vi "generate limit circle.vi"(8 "Radius Limit (mm)":dbl, 9 "Location Description":string, 10 "NewVal":T2 {"List of locations"."Position"."Position Y" format="%#.3f"; "List of locations"."Position"."Position X" format="%#.3f"}, 11 "Device Description":string) -> (2 "Center location":T1 {"Position"."Position Y" format="%#.3f"; "Position"."Position X" format="%#.3f"}, 3 "Circle":cluster{dbl[], dbl[]})   [LabVIEW 2017]
uses:
  device_list.ctl
  device.ctl
  location.ctl
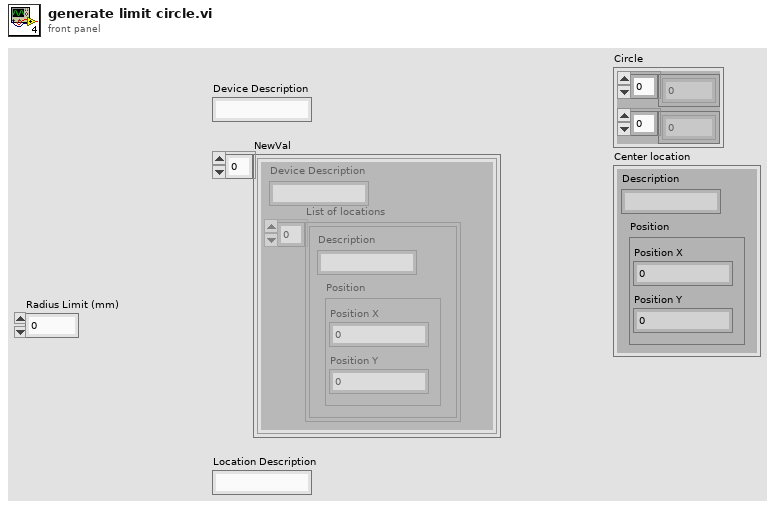
[diagram p1: front panel]
types:
  T1 = typedef "location.ctl" = cluster{"Description":string, "Position":cluster{"Position X":dbl, "Position Y":dbl}}
  T2 = typedef "device_list.ctl" = T3[]
  T3 = typedef "device.ctl" = cluster{"List of locations":T1[], "Device Description":string}
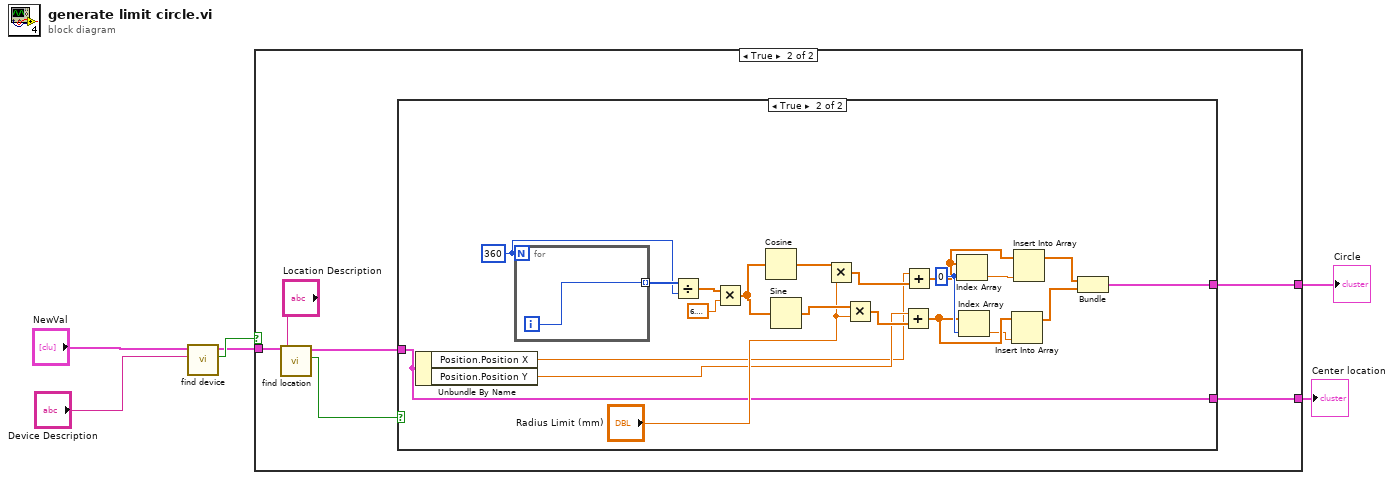
[diagram p0: block diagram]
diagram:
  n1 = call "find device.vi"("Device Description"="Device Description", "List of devices"="NewVal") -> ("Found?"=w6:bool, "Defualt Device"=w5:T3)  [unwired: 7 in, 1 out]
  n2 = case shown="True" w6 {
    tunnel: w5 -> [_ w12]
    tunnel: [_ w8] -> w2
    tunnel: [_ w7] -> w1
    frame False {
    }
    frame True {
      n3 = call "find location.vi"("Location Description"="Location Description", "Defualt Device"=w12) -> ("Found?"=w10:bool, "Location of input"=w9:T1)  [unwired: 7 in, 1 out]
      n4 = case shown="True" w10 {
        tunnel: w9 -> [_ w13]
        tunnel: [_ w15] -> w8
        tunnel: [_ w13] -> w7
        frame False {
        }
        frame True {
          w22 = 0 ("index")
          w27 = 360
          n5 = Unbundle By Name(w13) -> ("Position.Position X"=w14:dbl, "Position.Position Y"=w23:dbl)
          n6 = for {
            N: w27 -> [_]
            tunnel: [w34] -> w33 mode=indexing
            i -> [w34]
          }
          n7 = Divide(x=w33, y=w27) -> (x/y=w32:dbl[])
          n8 = Multiply(x=w32, y=6.283185307179586) -> (x*y=w31:dbl[])
          n9 = Cosine(x=w31) -> (cos(x)=w30:dbl[])
          n10 = Sine(x=w31) -> (sin(x)=w29:dbl[])
          n11 = Multiply(x=w30, y="Radius Limit (mm)") -> (x*y=w25:dbl[])
          n12 = Multiply(x=w29, y="Radius Limit (mm)") -> (x*y=w24:dbl[])
          n13 = Add(x=w23, y=w24) -> (x+y=w19:dbl[])
          n14 = Add(x=w14, y=w25) -> (x+y=w21:dbl[])
          n15 = Index Array(array=w21, index=w22) -> (element=w20:dbl)
          n16 = Index Array(array=w19, index=w22) -> (element=w18:dbl)
          n17 = Insert Into Array(array=w19, new element=w18) -> (w16:dbl[])  [unwired: 1 in]
          n18 = Insert Into Array(array=w21, new element=w20) -> (w17:dbl[])  [unwired: 1 in]
          n19 = Bundle(w17, w16) -> (w15:cluster{dbl[], dbl[]})  [unwired: 1 in]
        }
      }
    }
  }
  "Circle" <- w2
  "Center location" <- w1
